vi "Pulses_to_AgnleVel.vi"(11 "Encoder pulses":dbl) -> (1 "RPM":dbl, 2 "Deg/s":dbl, 3 "Rad/s":dbl)   [LabVIEW 2016]
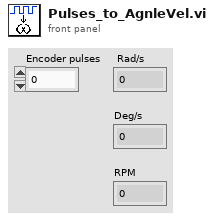
[diagram p1: front panel]
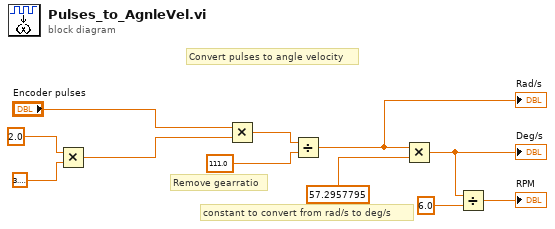
[diagram p0: block diagram]
diagram:
  # "Remove gearratio"
  # "constant to convert from rad/s to deg/s"
  # "Convert pulses to angle velocity"
  n1 = Multiply(x=2.0, y=3.141592653589793) -> (x*y=w3:dbl)
  n2 = Multiply(x="Encoder pulses", y=w3) -> (x*y=w4:dbl)
  n3 = Divide(x=w4, y=111.0) -> (x/y=w8:dbl)
  "Rad/s" <- w8
  n4 = Multiply(x=w8, y=57.2957795) -> (x*y=w11:dbl)
  "Deg/s" <- w11
  n5 = Divide(x=w11, y=6.0) -> (x/y=→"RPM":dbl)
